vi "Ordenar (SubVI).vi"(9 "Orden":bool, 10 "Columna":string="Fecha", 11 "Tabla":string="Tabla1") -> (3 "String":string)   [LabVIEW 2012]
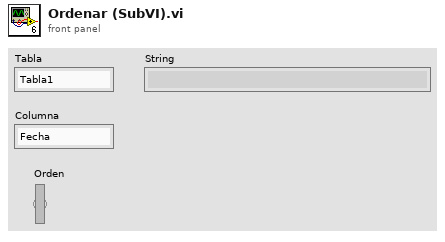
[diagram p1: front panel]
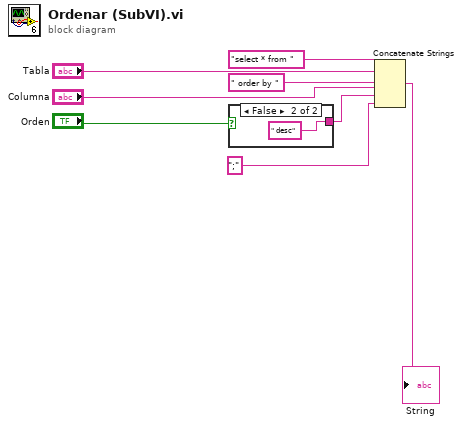
[diagram p0: block diagram]
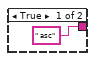
[diagram p2: hidden frame]
diagram:
  n1 = case shown="False" "Orden" {
    tunnel: [" asc" ("Substring") " desc" ("Substring")] -> w7
    frame True {
    }
    frame False {
    }
  }
  n2 = Concatenate Strings("select * from " ("SQL query"), "Tabla", " order by " ("Substring"), "Columna", w7, ";" ("Substring")) -> (→"String":string)
